vi "SCA.vi"(0 "System no.":i32=1 min=1 max=4 step=1, 2 "Axis 1":string, 3 "Axis 2":string, 5 "error in":errorcluster) -> (19 "error out":errorcluster)   [LabVIEW 2020]
doc: "Enables control of the two specified axes with controller keyboard cursor keys. Axis 1 can be controlled with left-right keys, axis 2 with up-down keys. The step width for each keystroke is set by SST.vi."
panel:
  # "Enables control of the two specified axes with\ncontroller keyboard cursor keys.  Axis 1 can be \ncontrolled with left right keys, axis 2 with up \ndown keys."
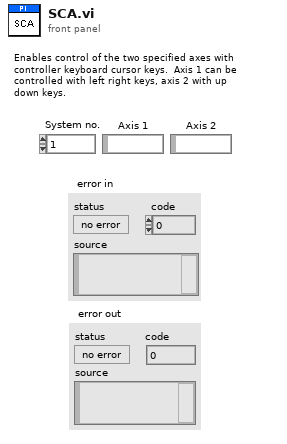
[diagram p1: front panel]
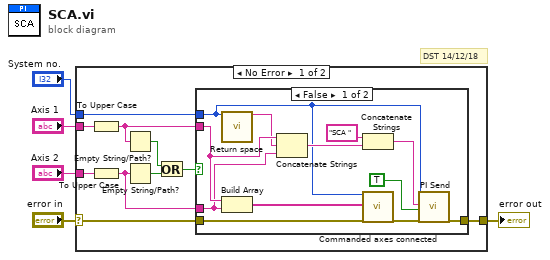
[diagram p0: block diagram]
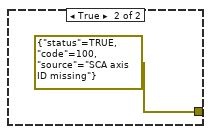
[diagram p2: hidden frame]
diagram:
  # "DST 14/12/18"
  n1 = case shown="No Error" "error in" {
    selector: "error in" -> [w10 w29]
    tunnel: "Axis 2" -> [w15 _]
    tunnel: "Axis 1" -> [w14 _]
    tunnel: "System no." -> [w13 _]
    tunnel: [w12 w29] -> w2
    frame No Error {
      n2 = To Upper Case(1:w14) -> (0:w8:string)
      n3 = To Upper Case(1:w15) -> (0:w7:string)
      n4 = Empty String/Path?(string/path=w8) -> (empty?=w9:bool)
      n5 = Empty String/Path?(string/path=w7) -> (empty?=w6:bool)
      n6 = Or(x=w9, y=w6) -> (x .or. y?=w11:bool)
      n7 = case shown="False" w11 {
        tunnel: w10 -> [w24 _]
        tunnel: w13 -> [w17 _]
        tunnel: [w21 errorcluster {"status"=TRUE, "code"=100, "source"="SCA axis ID missing"} ("error out")] -> w12
        tunnel: w8 -> [w19 _]
        tunnel: w7 -> [w18 _]
        frame False {
          n8 = call "Return space.vi"("System no."=w17) -> ("String out"=w16:string)  [unwired: 1 in, 17 out]
          n9 = Build Array(w19, w18) -> (w22:string[])
          n10 = Concatenate Strings(w19, w16, w18) -> (w20:string)
          n11 = Concatenate Strings("SCA ", w20) -> (w25:string)
          n12 = call "Commanded axes connected.vi"("System no."=w17, "Commanded axes"=w22, "error in"=w24) -> ("error out"=w23:errorcluster)  [unwired: 1 in, 15 out]
          n13 = call "PI Send.vi"("System no."=w17, "String to send"=w25, "Attach termination char.?"=TRUE ("Attach Linefeed?"), "error in"=w23) -> ("error out"=w21:errorcluster)  [unwired: 2 in, 13 out]
        }
        frame True {
        }
      }
    }
    frame Error {
    }
  }
  "error out" <- w2
